vi "Validate Lens Property.vi"(0 "Lens Property In":T1={"Unit"=TRUE, "Start "=1.0, "Stop "=1.0, "Dwell Time"=1.0, "Pause Time"=1.0, "Scans"=1, "Step Size"=1.0, "Row Numer"=0, "Ramp Time (ms)"=1, "Start DAC"=0, "Scan Type"=enum."Single"}, 1 "GUI Methode In":T3={"Lenses"=[], "Mass Ranges"=[], "Acquire"=FALSE, "MCA"=FALSE, "Q1DC EN"=FALSE, "Q1 POL"=FALSE, "Q3 POL"=FALSE, "Q1 RF  EN"=FALSE, "Averaging"=FALSE, "Log Scale"=FALSE, "CPS"=FALSE, "Units"=FALSE, "Data Path"=path "", "Run Mode"=enum."MRM (Q1/Q2)", "Fixed Mass (amu)"=1.0, "Q3DC EN"=FALSE, "Q3 RF  EN"=FALSE, "Negative"=FALSE} {"Mass Ranges"."Res" items=["High/High", "Medium/Medium", "Low/Low", "High/Medium", "High/Low", "Medium/High", "Medium/Low", "Low/High", "Low/Medium"]}, 2 "Error In":errorcluster) -> (3 "Lens Property Out":T1={"Unit"=TRUE, "Start "=1.0, "Stop "=1.0, "Dwell Time"=1.0, "Pause Time"=1.0, "Scans"=1, "Step Size"=1.0, "Row Numer"=0, "Ramp Time (ms)"=1, "Start DAC"=0, "Scan Type"=enum."Single"}, 4 "GUI Methode Out":T3={"Lenses"=[], "Mass Ranges"=[], "Acquire"=FALSE, "MCA"=FALSE, "Q1DC EN"=FALSE, "Q1 POL"=FALSE, "Q3 POL"=FALSE, "Q1 RF  EN"=FALSE, "Averaging"=FALSE, "Log Scale"=FALSE, "CPS"=FALSE, "Units"=FALSE, "Data Path"=path "", "Run Mode"=enum."MRM (Q1/Q2)", "Fixed Mass (amu)"=1.0, "Q3DC EN"=FALSE, "Q3 RF  EN"=FALSE, "Negative"=FALSE} {"Mass Ranges"."Res" items=["High/High", "Medium/Medium", "Low/Low", "High/Medium", "High/Low", "Medium/High", "Medium/Low", "Low/High", "Low/Medium"]}, 5 "Lens Table":string[][](table), 6 "Error Out":errorcluster)   [LabVIEW 2018]
uses:
  Type Defs/GUI Method.ctl
  Type Defs/Lenses.ctl
  GC-MSMSDevlopment/Type/_Mass Range Property.ctl
  GC-MSMSDevlopment/Type/_Mass Range Parameters.ctl
  GC-MSMSDevlopment/Type/_RT Res Type.ctl
  Type Defs/Run Mode.ctl
  Type Defs/Lens Property.ctl
  Type Defs/Scan Type.ctl
  Type Defs/Global Action.ctl
  Type Defs/State Machine.ctl
panel:
  in  "Units":bool
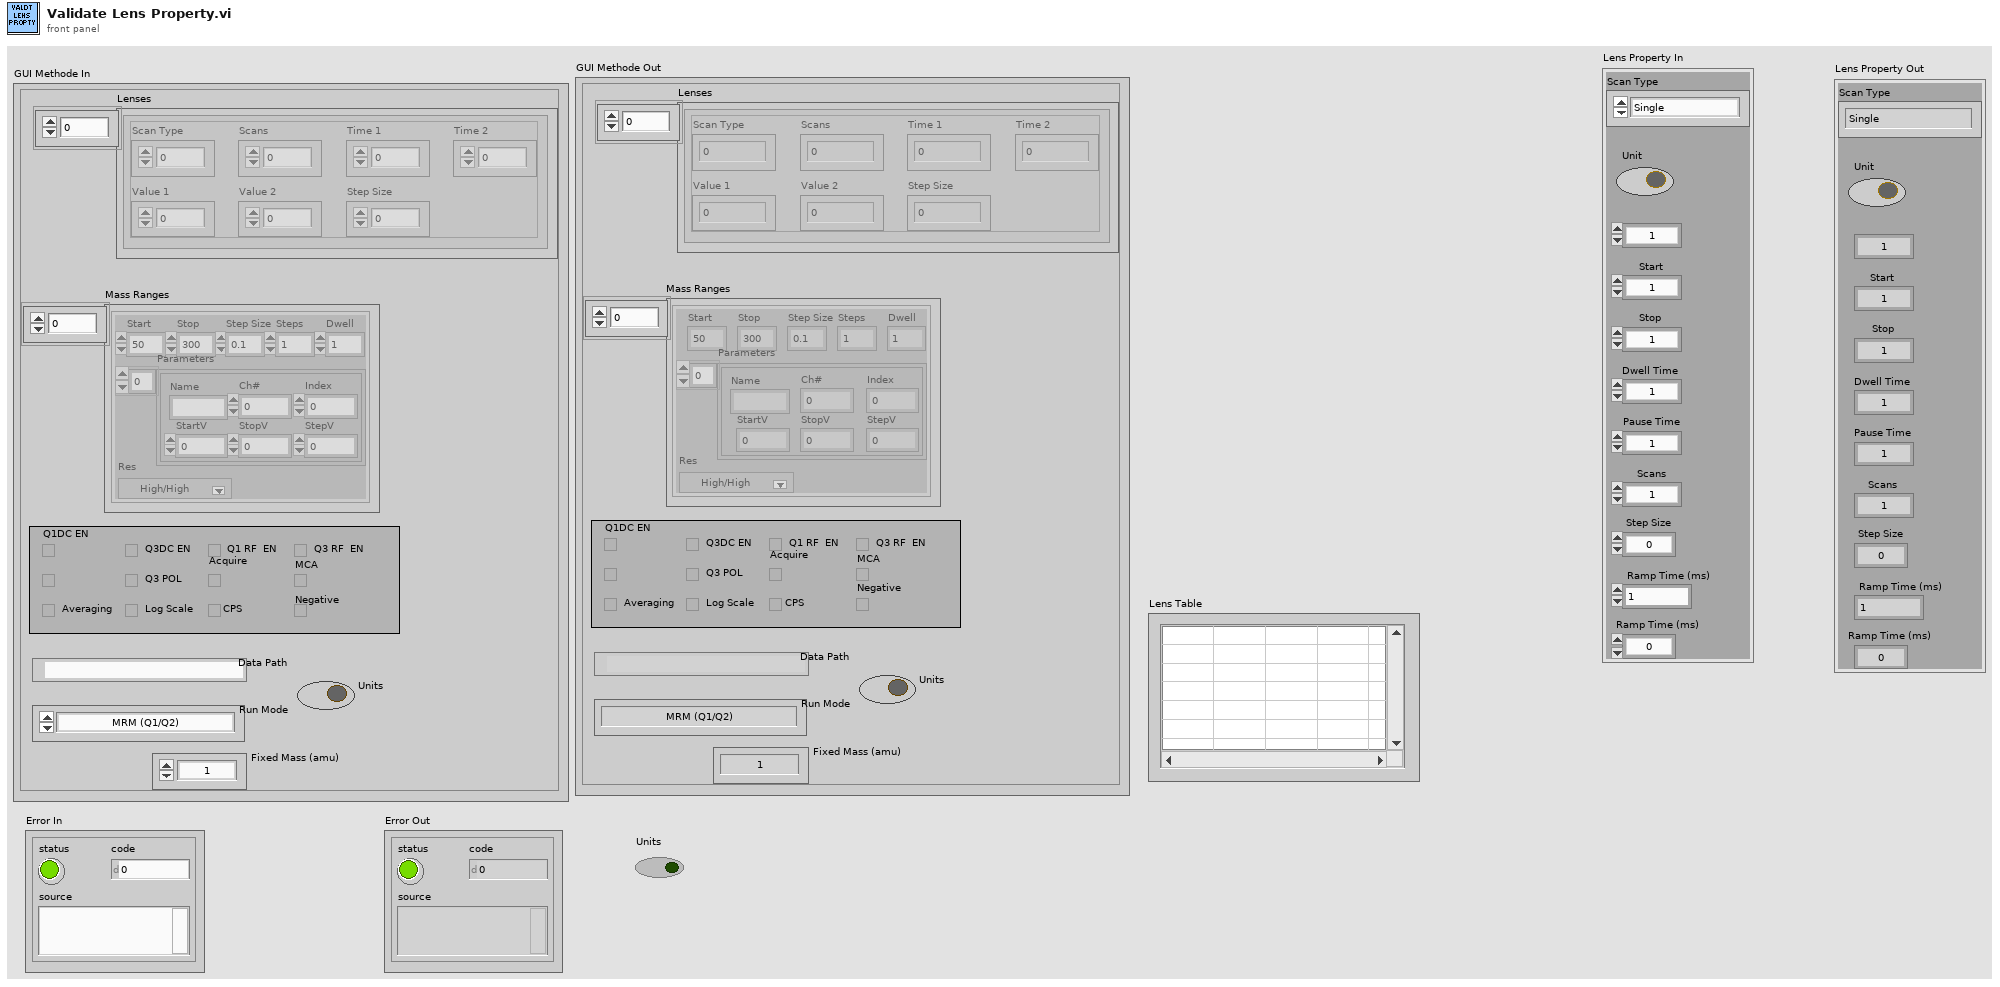
[diagram p1: front panel]
types:
  T1 = typedef "Lens Property.ctl" = cluster{"Unit":bool, "Start ":dbl, "Stop ":dbl, "Dwell Time":dbl, "Pause Time":dbl, "Scans":i32, "Step Size":dbl, "Row Numer":i32, "Ramp Time (ms)":i32, "Start DAC":i32, "Scan Type":T2}
  T2 = typedef "Scan Type.ctl" = enum8{"Single", "Dual", "Ramp"}
  T3 = typedef "GUI Method.ctl" = cluster{"Lenses":T4[], "Mass Ranges":T5[], "Acquire":bool, "MCA":bool, "Q1DC EN":bool, "Q1 POL":bool, "Q3 POL":bool, "Q1 RF  EN":bool, "Averaging":bool, "Log Scale":bool, "CPS":bool, "Units":bool, "Data Path":path, "Run Mode":T8, "Fixed Mass (amu)":dbl, "Q3DC EN":bool, "Q3 RF  EN":bool, "Negative":bool}
  T4 = typedef "Lenses.ctl" = cluster{"Scan Type":u8, "Scans":i32, "Time 1":dbl, "Time 2":dbl, "Value 1":dbl, "Value 2":dbl, "Step Size":dbl}
  T5 = typedef "_Mass Range Property.ctl" = cluster{"Start":dbl, "Stop":dbl, "Step Size":dbl, "Steps":i32, "Dwell":dbl, "Parameters":T6[], "Res":T7}
  T6 = typedef "_Mass Range Parameters.ctl" = cluster{"Name":string, "Ch#":u8, "StartV":dbl, "StopV":dbl, "StepV":dbl, "Index":u8}
  T7 = typedef "_RT Res Type.ctl" = u16
  T8 = typedef "Run Mode.ctl" = enum16{"MRM (Q1/Q2)", "Q1 Scan", "Q1 SRM", "Q2 Scan", "Q2 SRM", "Product Scan", "Precursor Scan", "Neutral Loss", "Neutral Gain"}
  T9 = typedef "State Machine.ctl" = enum16{"Case 0", "Case 1", "Case 2", "Case 3", "Case 4", "Case 5", "Case 6", "Case 7", "Case 8", "Case 9", "Case 10", "Error", "Exit"}
  T10 = typedef "Global Action.ctl" = enum16{"Write", "Read"}
  T11 = typedef "Global Configrations.ctl" = cluster{"Model Name":enum16{"QSight 110", "QSight 120", "QSight 210", "QSight 220", "QSight 410", "QSight 420", "IONICS 3Q 110", "IONICS 3Q 120", "IONICS 3Q 210", "IONICS 3Q 220", "IONICS 3Q 310", "IONICS 3Q 320", "Simulation (Single Source)", "Simulation (Dual Source)"}, "RunType":u16, "Acquisition State":enum16{"Ready", "Busy", "Waiting"}, "InstrState":enum16{"Initializing", "Mass Spectrometer is Off", "Starting Up", "Turning Power Off", "Going to Standby", "Roughing Pump Ready", "Turning Turbo Off", "Turbo Startup", "Turbopump Ready", "Checking Vacuum", "Going to Ready", "Ready", "Running", "Source Standby", "Lost Communication", "Shutting Down", "Fault", "24V Standby", "Go to 24V Standby", "Turbopump Ready-Waiting"}, "Run Mode":enum16{"MRM (Q1/Q2)", "Q1 Scan", "Q1 SRM", "Q2 Scan", "Q2 SRM", "Product Scan", "Precursor Scan", "Neutral Loss", "Neutral Gain"}, "Configration":T12, "TCP ID":refnum<k5>, "DT":bool, "Dead Time (nS)":i32, "Single Source":bool, "ADC Tables":T14[]}
  T12 = typedef "Configration.ctl" = cluster{"Table":T13[], "Instrument":string[]}
  T13 = typedef "_RT Configuration 2.ctl" = cluster{"Name":string, "Ch#":u8, "Min":dbl, "Max":dbl, "Def+":dbl, "Def-":dbl, "Offset":dbl, "Slope":dbl, "Type":u8, "Description":string, "SettleT":dbl}
  T14 = typedef "ADC Table.ctl" = cluster{"Name":string, "Ch#":u8, "Min":dbl, "Max":dbl, "Def+":dbl, "Def-":dbl, "Offset":dbl, "Slope":dbl, "Type":u8, "Description":string, "SettleT":dbl}
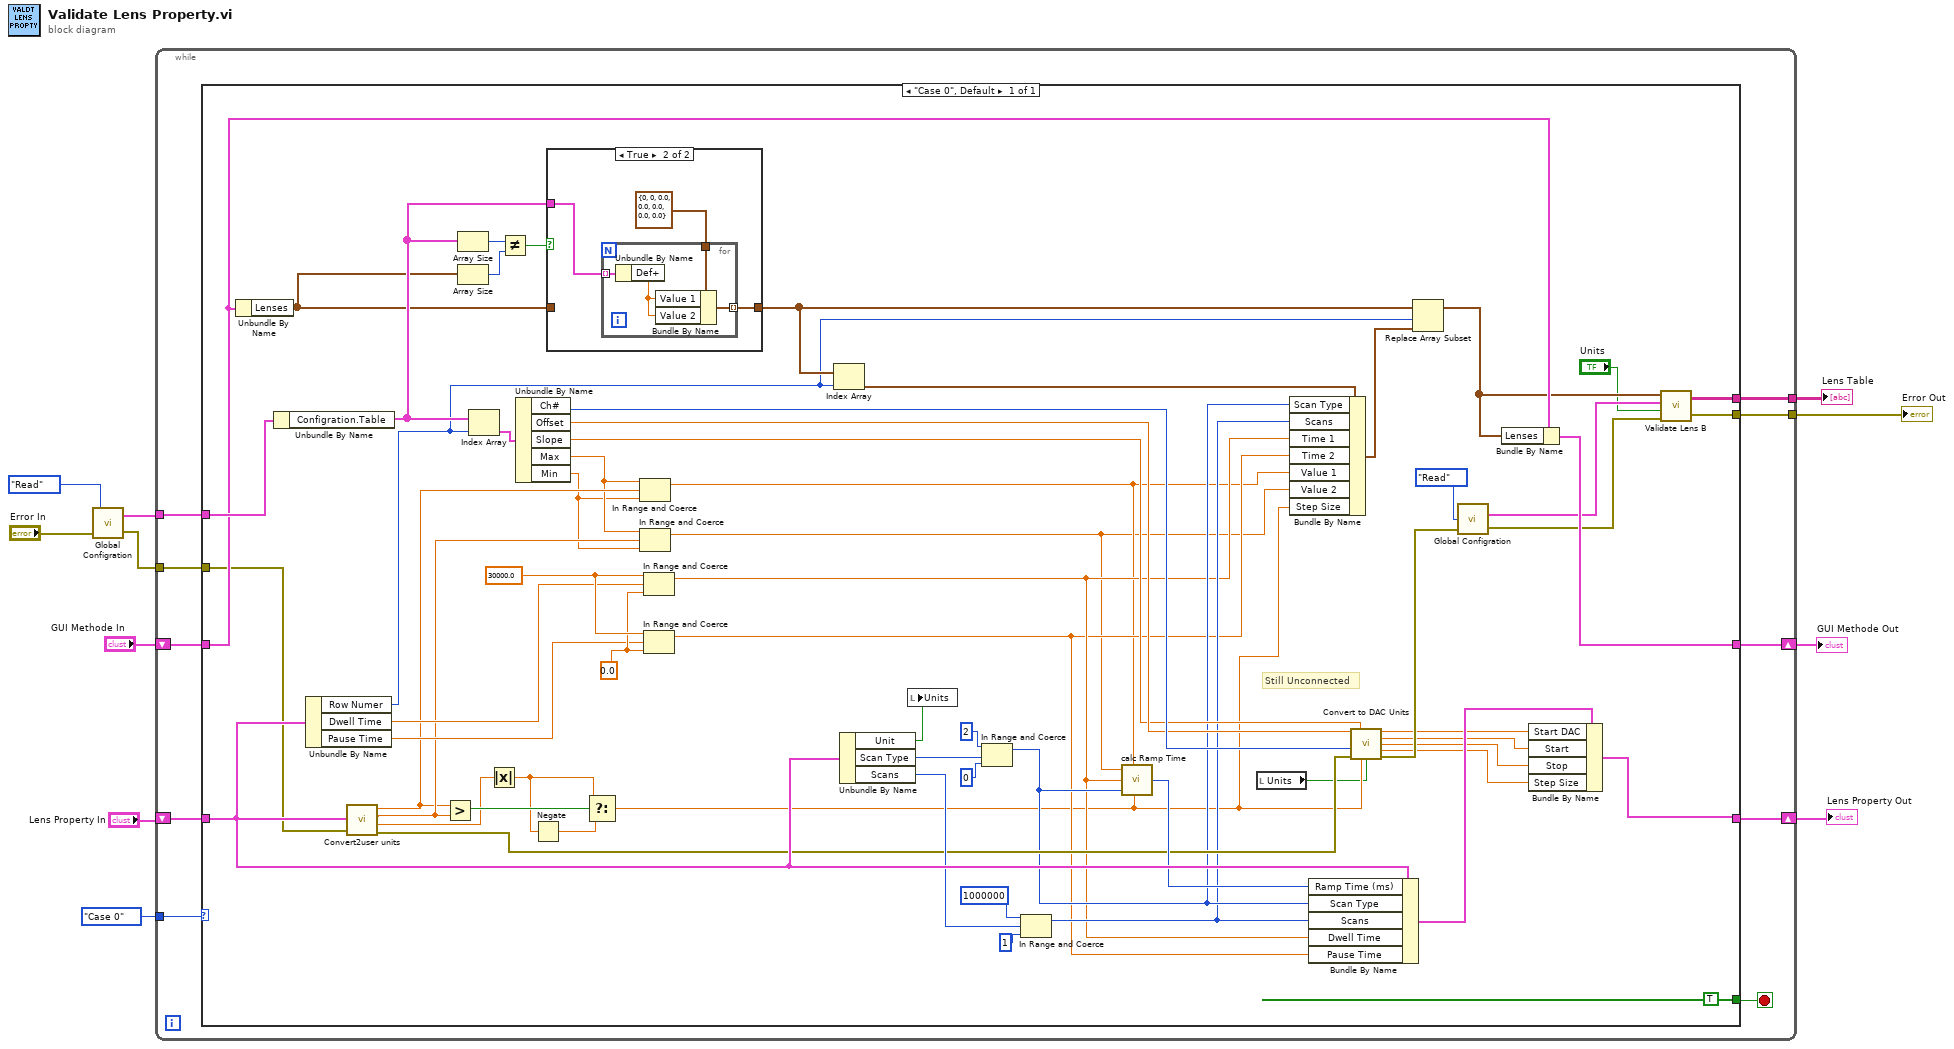
[diagram p0: block diagram]
diagram:
  n1 = call "Global Configration.vi"("Error In"="Error In", "Action"=Global_Action."Read") -> ("Error Out"=w5:errorcluster, "Parameters Out"=w6:T11)  [unwired: 1 in]
  n2 = while {
    shift-right: [w17] -> w4
    shift-left: "Lens Property In" -> [w19]
    shift-right: [w15] -> w3
    shift-left: "GUI Methode In" -> [w20]
    tunnel: w5 -> [w14]
    tunnel: [w13] -> w2
    tunnel: [w12] -> w1
    tunnel: w6 -> [w18]
    tunnel: State_Machine."Case 0" ("Enum") -> [w21]
    stop <- w16 stop-if-true
    n3 = case shown="\"Case 0\", Default" w21 {
      tunnel: w20 -> [w53]
      tunnel: w19 -> [w65]
      tunnel: w18 -> [w72]
      tunnel: [w38] -> w17
      tunnel: [TRUE] -> w16
      tunnel: [w52] -> w15
      tunnel: w14 -> [w50]
      tunnel: [w23] -> w12
      tunnel: [w22] -> w13
      frame "Case 0", Default {
        w78 = 0.0 ("lower limit")
        w79 = 30000.0 ("upper limit")
        # "Still Unconnected"
        n4 = Unbundle By Name(w53) -> ("Lenses"=w58:T4[])
        n5 = Unbundle By Name(w72) -> ("Configration.Table"=w60:T13[])
        n6 = Unbundle By Name(w65) -> ("Row Numer"=w54:i32, "Dwell Time"=w77:dbl, "Pause Time"=w76:dbl)
        n7 = call "Convert2user units.vi"("Lens Property In"=w65, "error in (no error)"=w50) -> ("OP 1"=w73:dbl, "OP 2"=w74:dbl, "OP 3"=w75:dbl, "error out"=w44:errorcluster)  [unwired: 1 in]
        n8 = Greater?(x=w73, y=w74) -> (0:w82:bool)
        n9 = Array Size(array=w60) -> (size(s)=w62:i32)
        n10 = Array Size(array=w58) -> (size(s)=w61:i32)
        n11 = Index Array(array=w60, index=w54) -> (element=w71:T13)
        n12 = Absolute Value(x=w75) -> (abs(x)=w80:dbl)
        n13 = Not Equal?(x=w62, y=w61) -> (x != y?=w59:bool)
        n14 = Unbundle By Name(w71) -> ("Ch#"=w49:u8, "Offset"=w46:dbl, "Slope"=w45:dbl, "Max"=w48:dbl, "Min"=w47:dbl)
        n15 = Negate(x=w80) -> (-x=w81:dbl)
        n16 = case shown="True" w59 {
          tunnel: [w84 w87] -> w55
          tunnel: w60 -> [_ w86]
          tunnel: w58 -> [w84 _]
          frame False {
          }
          frame True {
            n17 = for {
              tunnel: [w91] -> w87 mode=indexing
              tunnel: w86 -> [w89] mode=indexing
              tunnel: T4 {"Scan Type"=0, "Scans"=0, "Time 1"=0.0, "Time 2"=0.0, "Value 1"=0.0, "Value 2"=0.0, "Step Size"=0.0} ("Lenses") -> [w88]
              n18 = Unbundle By Name(w89) -> ("Def+"=w90:dbl)
              n19 = Bundle By Name(cluster=w88, "Value 1"=w90, "Value 2"=w90) -> (w91:T4)
            }
          }
        }
        n20 = Select(t=w80, s=w82, f=w81) -> (s? t:f=w30:dbl)
        n21 = In Range and Coerce(upper limit=w48, x=w73, lower limit=w47) -> (coerced(x)=w32:dbl)  [unwired: 1 out]
        n22 = In Range and Coerce(upper limit=w48, x=w74, lower limit=w47) -> (coerced(x)=w31:dbl)  [unwired: 1 out]
        n23 = In Range and Coerce(upper limit=w79, x=w77, lower limit=w78) -> (coerced(x)=w34:dbl)  [unwired: 1 out]
        n24 = In Range and Coerce(upper limit=w79, x=w76, lower limit=w78) -> (coerced(x)=w33:dbl)  [unwired: 1 out]
        n25 = Index Array(array=w55, index=w54) -> (element=w57:T4)
        n26 = Unbundle By Name(w65) -> ("Unit"=w25:bool, "Scan Type"=w67:T2, "Scans"=w63:i32)
        n27 = local write "Units"(w25) -> ()
        n28 = In Range and Coerce(upper limit=u8 2, x=w67, lower limit=u8 0) -> (coerced(x)=w36:u8)  [unwired: 1 out]
        n29 = In Range and Coerce(upper limit=1000000, x=w63, lower limit=1) -> (coerced(x)=w35:i32)  [unwired: 1 out]
        n30 = call "calc Ramp Time.vi"("Stop"=w31, "Start"=w32, "Dwell (ms)"=w34, "Scan Type"=w36, "Step"=w30) -> ("Ramp Time (ms)"=w64:i32)
        n31 = local read "Units"() -> (w24:bool)
        n32 = Bundle By Name(cluster=w57, "Scan Type"=w36, "Scans"=w35, "Time 1"=w34, "Time 2"=w33, "Value 1"=w32, "Value 2"=w31, "Step Size"=w30) -> (w56:T4)
        n33 = Bundle By Name(cluster=w65, "Ramp Time (ms)"=w64, "Scan Type"=w36, "Scans"=w35, "Dwell Time"=w34, "Pause Time"=w33) -> (w42:T1)
        n34 = call "Convert to DAC Units.vi"("Offset"=w46, "Slope"=w45, "Ch#"=w49, "error in (no error)"=w44, "s? t:f"=w30, "Units"=w24) -> ("OP 1"=w41:dbl, "OP 2"=w37:dbl, "OP 3"=w39:dbl, "OP 4"=w40:dbl, "error out"=w43:errorcluster)  [unwired: 5 in]
        n35 = Replace Array Subset(array=w55, new element=w56, index=w54) -> (w29:T4[])
        n36 = call "Global Configration.vi"("Error In"=w43, "Action"=Global_Action."Read") -> ("Error Out"=w27:errorcluster, "Parameters Out"=w28:T11)  [unwired: 1 in]
        n37 = Bundle By Name(cluster=w53, "Lenses"=w29) -> (w52:T3)
        n38 = Bundle By Name(cluster=w42, "Start DAC"=w41, "Start"=w37, "Stop"=w39, "Step Size"=w40) -> (w38:T1)
        n39 = call "Validate Lens B.vi"("Error In"=w27, "Units"="Units", "Parameters In"=w28, "Lenses"=w29) -> ("Error Out"=w23:errorcluster, "Lens Table"=w22:string[][])
      }
    }
  }
  "GUI Methode Out" <- w3
  "Lens Table" <- w2
  "Error Out" <- w1
  "Lens Property Out" <- w4
